vi "selectAutonMode.vi"(1 "Joystick":bool) -> ()   [LabVIEW 2011]
uses:
  <vilib>/Rock Robotics/WPI/DriverStation/DriverStationLCD/WPI_DriverStationLCDLCDLine.ctl
  Robot Global Data.vi
panel:
  in  "File Number":dbl
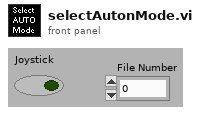
[diagram p1: front panel]
types:
  T1 = typedef "WPI_DriverStationLCDLCDLine.ctl" = enum16{"Main - Line 1", "User - Line 2", "User - Line 3", "User - Line 4", "User - Line 5", "User - Line 6"}
  T2 = enum16{"False", "FalseToTrue", "True", "TrueToFalse"}
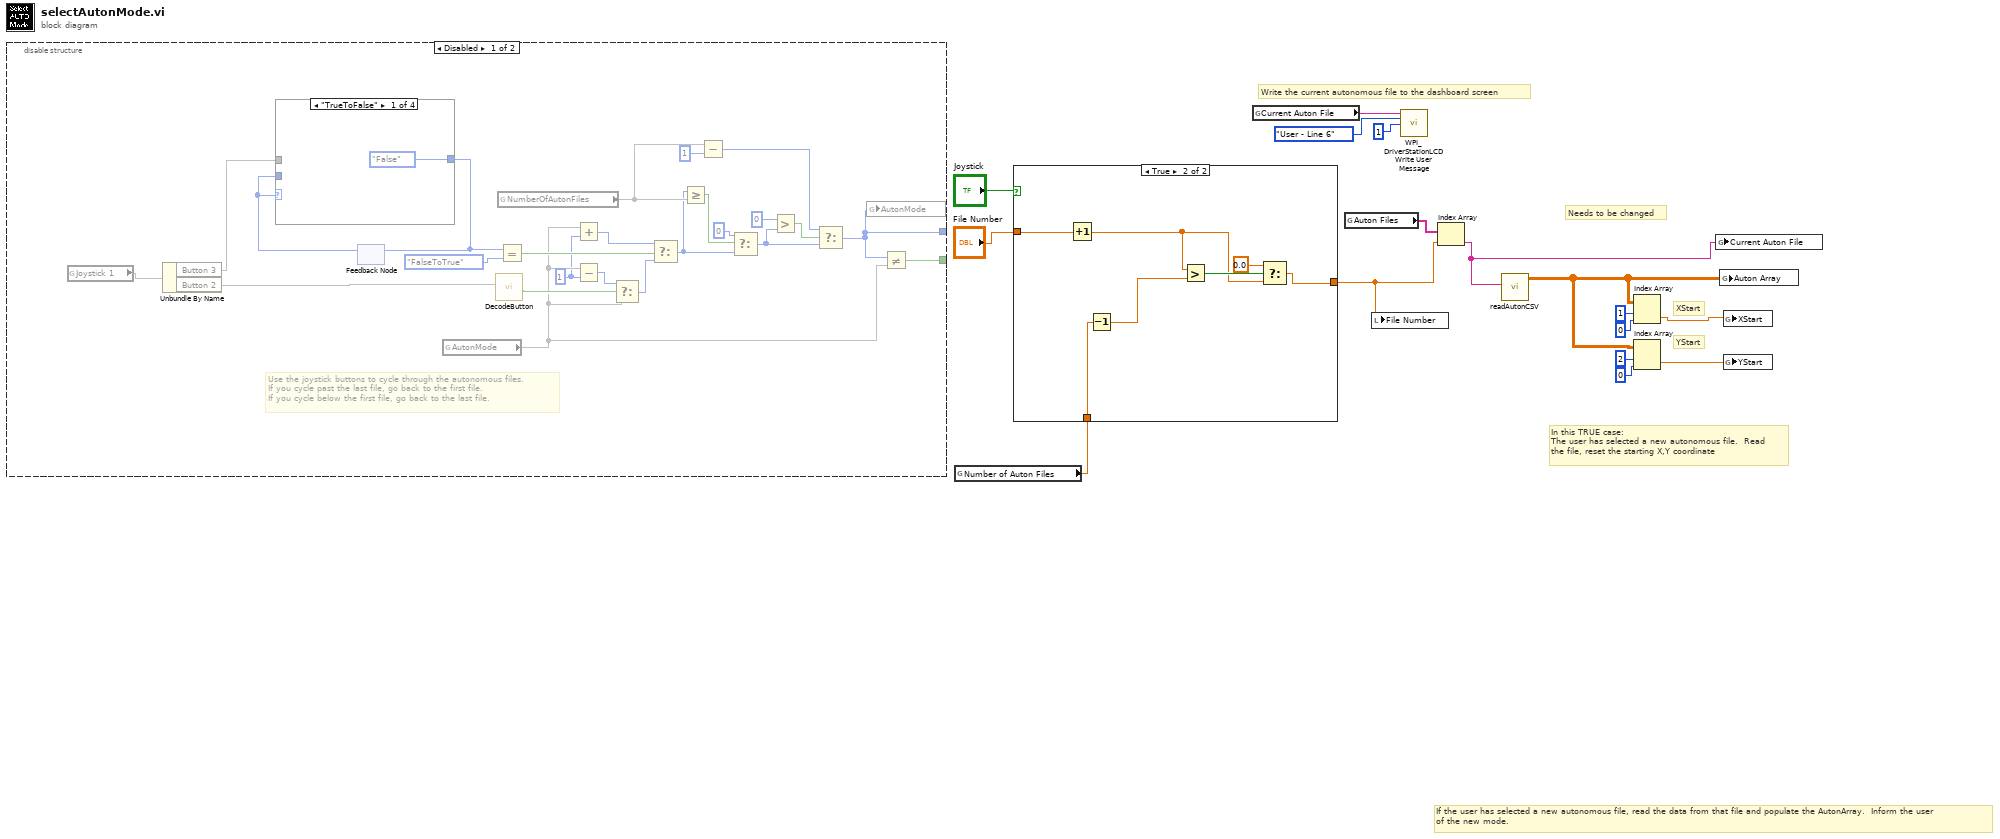
[diagram p0: block diagram]
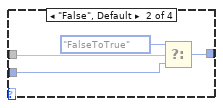
[diagram p3: hidden frame]
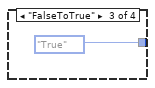
[diagram p4: hidden frame]
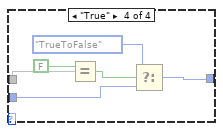
[diagram p5: hidden frame]
diagram:
  # "Needs to be changed"
  # "In this TRUE case:\nThe user has selected a new autonomous file.  Read\nthe file, reset the starting X,Y coordinate"
  # "YStart"
  # "XStart"
  # "Write the current autonomous file to the dashboard screen"
  # "If the user has selected a new autonomous file, read the data from that file and populate the AutonArray.  Inform the user\nof the new mode."
  n1 = disable-structure shown="Disabled" {
    disable-tunnel: [w40 _] -> _
    disable-tunnel: [w30 _] -> _
    frame Disabled {
      w21 = i16 1 ("y")
      # "Use the joystick buttons to cycle through the autonomous files.\nIf you cycle past the last file, go back to the first file.\nIf you cycle below the first file, go back to the last file."
      n2 = global read "Robot Global Data.vi" "Joystick 1"() -> (w17)
      n3 = Unbundle By Name(w17) -> ("Button 3"=w28, "Button 2"=w18)
      n4 = feedback #1() -> (w25:T2)  [unwired: 1 out]
      n5 = case shown="\"TrueToFalse\"" w25 {
        tunnel: w28 -> [_ w45 _ w51]
        tunnel: [T2."False" ("f") w43 T2."True" ("y") w52] -> w26
        tunnel: w25 -> [_ w42 _ w48]
        frame "TrueToFalse" {
        }
        frame "False", Default {
          n6 = Select(t=T2."FalseToTrue", s=w45, f=w42) -> (s? t:f=w43:T2)
        }
        frame "FalseToTrue" {
        }
        frame "True" {
          n7 = Equal?(x=FALSE, y=w51) -> (x = y?=w49:bool)
          n8 = Select(t=T2."TrueToFalse", s=w49, f=w48) -> (s? t:f=w52:T2)
        }
      }
      n9 = feedback-in #1(w26) -> ()
      n10 = global read "Robot Global Data.vi" "AutonMode"() -> (w23)
      n11 = call "DecodeButton.vi"("Button"=w18) -> ("False to True"=w24:bool)  [unwired: 10 out]
      n12 = global read "Robot Global Data.vi" "NumberOfAutonFiles"() -> (w37)
      n13 = Equal?(x=w26, y=T2."FalseToTrue") -> (x = y?=w29:bool)
      n14 = Add(x=w23, y=w21) -> (x+y=w22:i16)
      n15 = Subtract(x=w23, y=w21) -> (x-y=w19:i16)
      n16 = Select(t=w19, s=w24, f=w23) -> (s? t:f=w20:i16)
      n17 = Select(t=w22, s=w29, f=w20) -> (s? t:f=w31:i16)
      n18 = Greater Or Equal?(x=w31, y=w37) -> (x >= y?=w32:bool)
      n19 = Subtract(x=w37, y=i16 1) -> (x-y=w39:i16)
      n20 = Select(t=i16 0, s=w32, f=w31) -> (s? t:f=w34:i16)
      n21 = Greater?(x=i16 0, y=w34) -> (0:w36:bool)
      n22 = Select(t=w39, s=w36, f=w34) -> (s? t:f=w40:i16)
      n23 = global write "Robot Global Data.vi" "AutonMode"(w40) -> ()
      n24 = Not Equal?(x=w40, y=w23) -> (x != y?=w30:bool)
    }
    frame Enabled {
    }
  }
  n25 = global read "Robot Global Data.vi" "Number of Auton Files"() -> (w8:dbl)
  n26 = case shown="True" "Joystick" {
    tunnel: "File Number" -> [w53 w60]
    tunnel: [w53 w56] -> w7
    tunnel: w8 -> [_ w55]
    frame False {
    }
    frame True {
      n27 = Increment(x=w60) -> (x+1=w58:dbl)
      n28 = Decrement(x=w55) -> (x-1=w54:dbl)
      n29 = Greater?(x=w58, y=w54) -> (0:w59:bool)
      n30 = Select(t=0.0, s=w59, f=w58) -> (s? t:f=w56:dbl)
    }
  }
  n31 = global read "Robot Global Data.vi" "Current Auton File"() -> (w6:string)
  n32 = global read "Robot Global Data.vi" "Auton Files"() -> (w5:string[])
  n33 = local write "File Number"(w7) -> ()
  n34 = call <vilib>:"WPI_DriverStationLCDWrite User Message.vi"("line text"=w6, "line"=WPI_DriverStationLCDLCDLine."User - Line 6", "starting column"=i8 1) -> ()  [unwired: 2 in, 11 out]
  n35 = Index Array(array=w5, index=w7) -> (element=w1:string)
  n36 = call "readAutonCSV.vi"("AutonFile"=w1) -> ("AutonArray"=w4:dbl[][])  [unwired: 7 out]
  n37 = Index Array(array=w4, index (row)=1 ("disabled index (row)"), index (col)=0) -> (element=w3:dbl)
  n38 = Index Array(array=w4, index (row)=2 ("disabled index (row)"), index (col)=0) -> (element=w2:dbl)
  n39 = global write "Robot Global Data.vi" "Current Auton File"(w1) -> ()
  n40 = global write "Robot Global Data.vi" "Auton Array"(w4) -> ()
  n41 = global write "Robot Global Data.vi" "XStart"(w3) -> ()
  n42 = global write "Robot Global Data.vi" "YStart"(w2) -> ()
